vi "Event Selector.vi"(8 "Error In":errorcluster, 9 "Session In":T3="cam0", 10 "Pass In Event":bool, 11 "Manual Pass In Event":T1=enum."Start Button Pressed") -> (0 "Error Out":errorcluster, 1 "Session Out":T3="cam0", 3 "Event Queue":T1[](array[typedef]))   [LabVIEW 2017]
uses:
  <vilib>/userdefined/High Color/IMAQdx.ctl
  state-manager/Event.ctl
  Sense/Camera/Colour Typedef.ctl
  <vilib>/myRIO/Instrument Drivers/Onboard IO/DIO/typedefs/DIO Reference.ctl
  <vilib>/myRIO/Common/Instrument Driver Framework/Utilities/typedefs/myRIO Generic Hardware Reference.ctl
  <vilib>/myRIO/Common/Instrument Driver Framework/Utilities/typedefs/Hardware Version Enum.ctl
  <vilib>/myRIO/Common/Instrument Driver Framework/Utilities/typedefs/myRIO v1.0 Reference.ctl
  <vilib>/myRIO/Common/Instrument Driver Framework/Utilities/typedefs/Generic FPGA Reference.ctl
  <vilib>/myRIO/Common/Instrument Driver Framework/myRIO v1.0/DIO/typedefs/DIO Channels List.ctl
  <vilib>/myRIO/Common/Instrument Driver Framework/myRIO v1.0/DIO/typedefs/DIO Channels Enum.ctl
  <vilib>/userdefined/High Color/nirio_resource_hc.ctl
  <vilib>/myRIO/Common/Instrument Driver Framework/Utilities/vis/Is FPGA Ref Available.vi
  <vilib>/myRIO/Common/Instrument Driver Framework/myRIO v1.0/DIO/vis/myRIO v1.1 Open DIO.vi
  <vilib>/myRIO/Instrument Drivers/Onboard IO/DIO/vis/Read.vi
  <vilib>/myRIO/Common/Instrument Driver Framework/Utilities/vis/Validate Channels.vi
  <vilib>/myRIO/Common/Instrument Driver Framework/myRIO v1.0/DIO/vis/myRIO v1.0 Reserve DIO.vi
  <vilib>/myRIO/Common/Instrument Driver Framework/myRIO v1.0/Resource Manager/vis/myRIO v1.0 Reserve Channel List.vi
  <vilib>/myRIO/Common/Instrument Driver Framework/myRIO v1.0/DIO/vis/myRIO v1.0 Build MUX Configuration DIO.vi
  <vilib>/myRIO/Common/Instrument Driver Framework/myRIO v1.0/Resource Manager/vis/myRIO v1.0 Reserve Channel.vi
  <vilib>/myRIO/Common/Instrument Driver Framework/myRIO v1.0/Resource Manager/vis/myRIO v1.0 Unreserve Channel.vi
  <vilib>/myRIO/Common/Instrument Driver Framework/myRIO v1.0/Resource Manager/vis/myRIO v1.0 Create Configuration List.vi
  <vilib>/myRIO/Common/Instrument Driver Framework/myRIO v1.0/Resource Manager/vis/myRIO v1.0 Build Mutex Name.vi
  Globals/Pose.vi
  <vilib>/Utility/VariantDataType/GetNumericInfo.vi
  <vilib>/Utility/error.llb/Error Cluster From Error Code.vi
  <vilib>/myRIO/Common/Instrument Driver Framework/myRIO v1.0/myRIO v1.1 Open.vi
  <vilib>/myRIO/Common/Instrument Driver Framework/Utilities/vis/IO Manager.vi
  <vilib>/myRIO/Common/Instrument Driver Framework/Utilities/vis/Configuration Manager.vi
  <vilib>/myRIO/Common/Instrument Driver Framework/myRIO v1.0/Resource Manager/vis/myRIO v1.0 Configure IO.vi
  <vilib>/myRIO/Common/Instrument Driver Framework/myRIO v1.0/myRIO v1.0 Close.vi
  <vilib>/myRIO/Common/Instrument Driver Framework/myRIO v1.0/DIO/vis/myRIO v1.0 Read DIO.vi
  Globals/Zig Zag Global.vi
  <vilib>/myRIO/Express VI/Onboard IO/DI/DI Express VI.xnode
  <vilib>/myRIO/Instrument Drivers/Onboard IO/DIO/vis/myRIO DIO Open.xnode
  <vilib>/myRIO/Instrument Drivers/Onboard IO/DIO/DIO.lvlib
panel:
  out "Line Colour":T2=enum."None"
  out "Line Color Confidence (0-100)":dbl=99.98833333333333
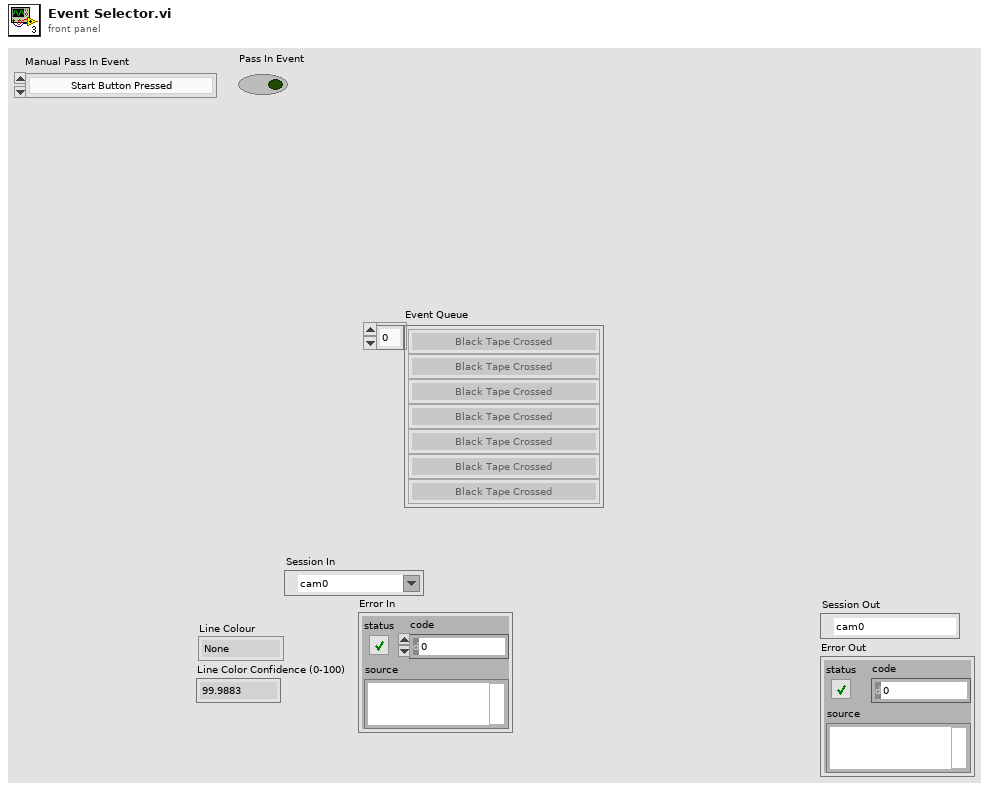
[diagram p1: front panel]
types:
  T1 = typedef "Event.ctl" = enum16{"None", "Zig Zag Finished", "Start Obstacle Avoidance", "Start Button Pressed", "Black & Yellow Tape Touched", "Black & Yellow Tape Passed", "Green Tape Crossed", "Red Tape Touched", "Rough Terrain Touched", "Black Tape Crossed", "Tape Edge Too Close", "Wall Too Close", "Rough Terrain Passed", "Ramp Passed", "Stop Button Pressed", "Recentered", "End Zone Wait Timed Out"}
  T2 = typedef "Colour Typedef.ctl" = enum16{"Yellow", "Red", "Black", "Green", "Blue", "None", "Black&Yellow"}
  T3 = typedef "IMAQdx.ctl" = refnum<k21>
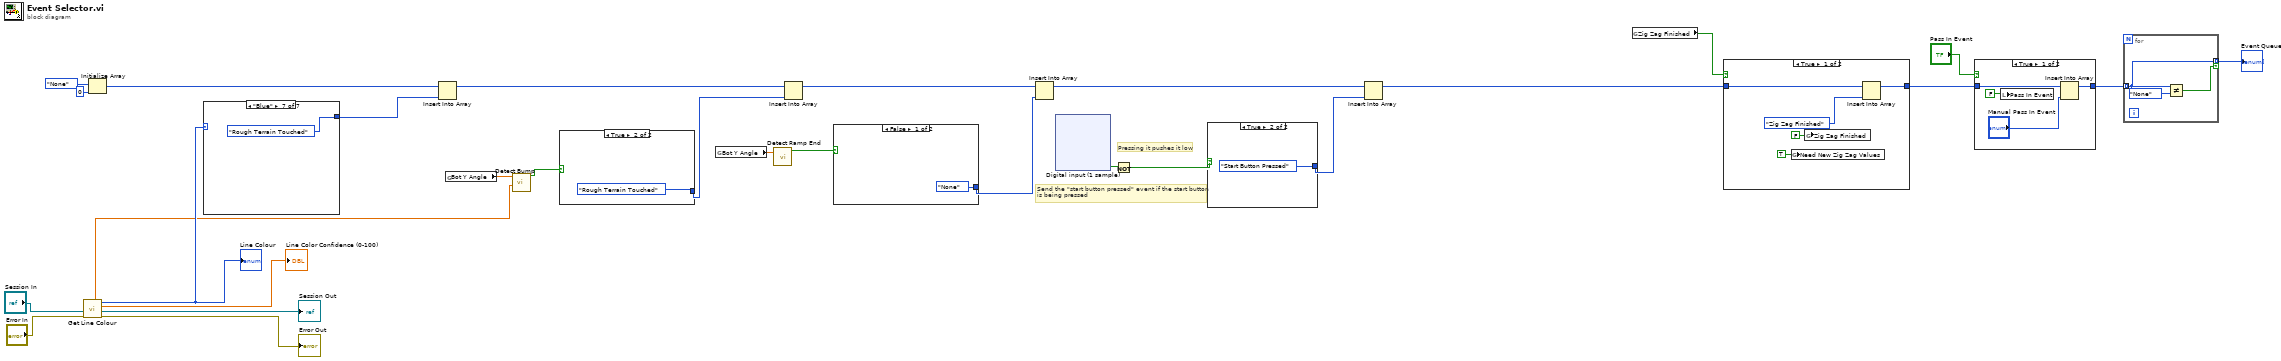
[diagram p0: block diagram]
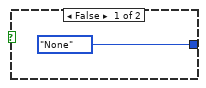
[diagram p3: hidden frame]
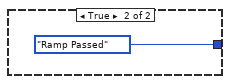
[diagram p4: hidden frame]
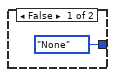
[diagram p5: hidden frame]
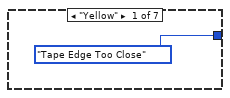
[diagram p7: hidden frame]
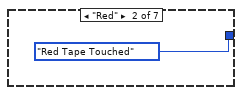
[diagram p8: hidden frame]
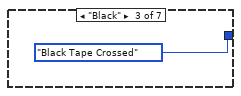
[diagram p9: hidden frame]
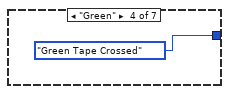
[diagram p10: hidden frame]
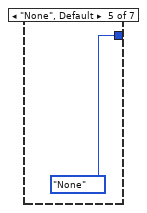
[diagram p11: hidden frame]
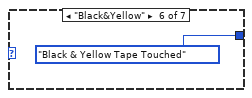
[diagram p12: hidden frame]
diagram:
  # "Pressing it pushes it low"
  # "Send the \"start button pressed\" event if the start button\nis being pressed"
  n1 = call "Get Line Colour.vi"("Error In"="Error In", "Session In"="Session In") -> ("Error Out"=→"Error Out":errorcluster, "Session Out"=→"Session Out":T3, "Confidence (0-100)"=→"Line Color Confidence (0-100)":dbl, "Colour"=w23:T2, "Blue"=w21:dbl)  [unwired: 5 in]
  "Line Colour" <- w23
  n2 = Initialize Array(Event."None" ("Event 2"), 0 ("dimension size")) -> (w8:T1[])
  n3 = case shown="\"Blue\"" w23 {
    tunnel: [Event."Tape Edge Too Close" ("Event 2") Event."Red Tape Touched" ("Event 2") Event."Black Tape Crossed" ("Event 2") Event."Green Tape Crossed" ("Event 2") Event."None" ("Event 2") Event."Black & Yellow Tape Touched" ("Event 2") Event."Rough Terrain Touched" ("Event 2")] -> w18
    frame "Yellow" {
    }
    frame "Red" {
    }
    frame "Black" {
    }
    frame "Green" {
    }
    frame "None", Default {
    }
    frame "Black&Yellow" {
    }
    frame "Blue" {
    }
  }
  n4 = Insert Into Array(array=w8, new element=w18) -> (w17:T1[])  [unwired: 1 in]
  n5 = global read "Pose.vi" "Bot Y Angle"() -> (w19:dbl)
  n6 = call "Detect Bump.vi"("Blue Confidence"=w21, "y angle"=w19) -> ("Bumpy Terrain"=w22:bool)  [unwired: 9 in]
  n7 = case shown="True" w22 {
    tunnel: [Event."None" ("Event 2") Event."Rough Terrain Touched" ("Event 2")] -> w16
    frame False {
    }
    frame True {
    }
  }
  n8 = global read "Pose.vi" "Bot Y Angle"() -> (w9:dbl)
  n9 = call "Detect Ramp End.vi"("y angle"=w9) -> ("Ramp Just Ended"=w20:bool)  [unwired: 10 in]
  n10 = Insert Into Array(array=w17, new element=w16) -> (w15:T1[])  [unwired: 1 in]
  n11 = case shown="False" w20 {
    tunnel: [Event."None" ("Event 2") Event."Ramp Passed" ("Event 2")] -> w14
    frame False {
    }
    frame True {
    }
  }
  n12 = Insert Into Array(array=w15, new element=w14) -> (w12:T1[])  [unwired: 1 in]
  n13 = xnode "Digital input (1 sample)"() -> ("A/DIO1 (Pin 13)"=w25:bool)  [unwired: 1 in, 1 out]
  n14 = Not(x=w25) -> (.not. x?=w13:bool)
  n15 = case shown="True" w13 {
    tunnel: [Event."None" ("Event 2") Event."Start Button Pressed" ("Event 2")] -> w11
    frame False {
    }
    frame True {
    }
  }
  n16 = Insert Into Array(array=w12, new element=w11) -> (w1:T1[])  [unwired: 1 in]
  n17 = global read "Zig Zag Global.vi" "Zig Zag Finished"() -> (w2:bool)
  n18 = case shown="True" w2 {
    tunnel: w1 -> [w47 w48]
    tunnel: [w46 w48] -> w3
    frame True {
      n19 = global write "Zig Zag Global.vi" "Need New Zig Zag Values"(TRUE ("Need New Zig Zag Values")) -> ()
      n20 = global write "Zig Zag Global.vi" "Zig Zag Finished"(FALSE ("Zig Zag Finished")) -> ()
      n21 = Insert Into Array(array=w47, new element=Event."Zig Zag Finished" ("Event 2")) -> (w46:T1[])  [unwired: 1 in]
    }
    frame False {
    }
  }
  n22 = case shown="True" "Pass In Event" {
    tunnel: w3 -> [w51 w53]
    tunnel: [w49 w53] -> w4
    frame True {
      n23 = local write "Pass In Event"(FALSE ("Pass In Event")) -> ()
      n24 = Insert Into Array(array=w51, new element="Manual Pass In Event") -> (w49:T1[])  [unwired: 1 in]
    }
    frame False {
    }
  }
  n25 = for {
    tunnel: [w54] -> w5 mode=indexing if=w55
    tunnel: w4 -> [w54] mode=indexing
    n26 = Not Equal?(x=w54, y=Event."None") -> (x != y?=w55:bool)
  }
  "Event Queue" <- w5
